vi "jk-flip-flop.vi"(9 "K in":bool, 10 "CLK":bool, 11 "J":bool) -> (2 "!Q":bool, 3 "Q":bool)   [LabVIEW 2024]
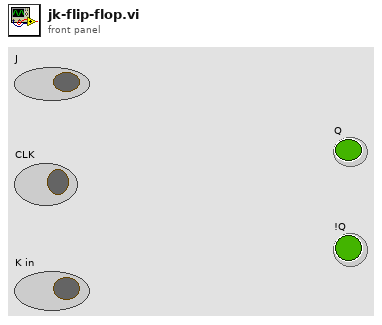
[diagram p1: front panel]
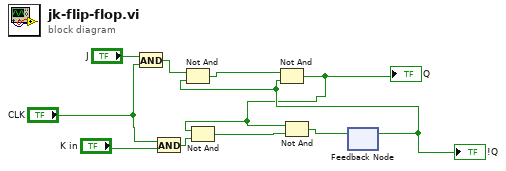
[diagram p0: block diagram]
diagram:
  n1 = And(x="J", y="CLK") -> (x .and. y?=w1:bool)
  n2 = And(x="CLK", y="K in") -> (x .and. y?=w3:bool)
  n3 = feedback #1() -> (w10:bool)  [unwired: 1 in]
  "!Q" <- w10
  n4 = Not And(1:w10, 2:w1) -> (0:w6:bool)
  n5 = Not And(1:w10, 2:w6) -> (0:w9:bool)
  "Q" <- w9
  n6 = Not And(1:w3, 2:w9) -> (0:w7:bool)
  n7 = Not And(1:w7, 2:w9) -> (0:w8:bool)
  n8 = feedback-in #1(w8) -> ()
